vi "AppendEventInfoH5.vi"(6 "evt_num":i32, 8 "error in (no error)":errorcluster, 9 "evt_time":dbl, 10 "TDC Data":u32[](array[numeric]), 11 "dset in":T2 format="%.0x") -> (0 "error out":errorcluster)   [LabVIEW 2014]
uses:
  <vilib>/addons/h5labview2/base/hid_t.ctl
  <vilib>/addons/h5labview2/base/lib_path.vi
  <vilib>/addons/h5labview2/base/H5Equery.vi
  <vilib>/addons/h5labview2/dataset/H5Dwrite.llb/H5Dwrite.xnode
  <vilib>/addons/h5labview2/dataset/H5D.lvlib
  <vilib>/addons/h5labview2/space/H5S.lvlib
panel:
  in  "Cluster":T1
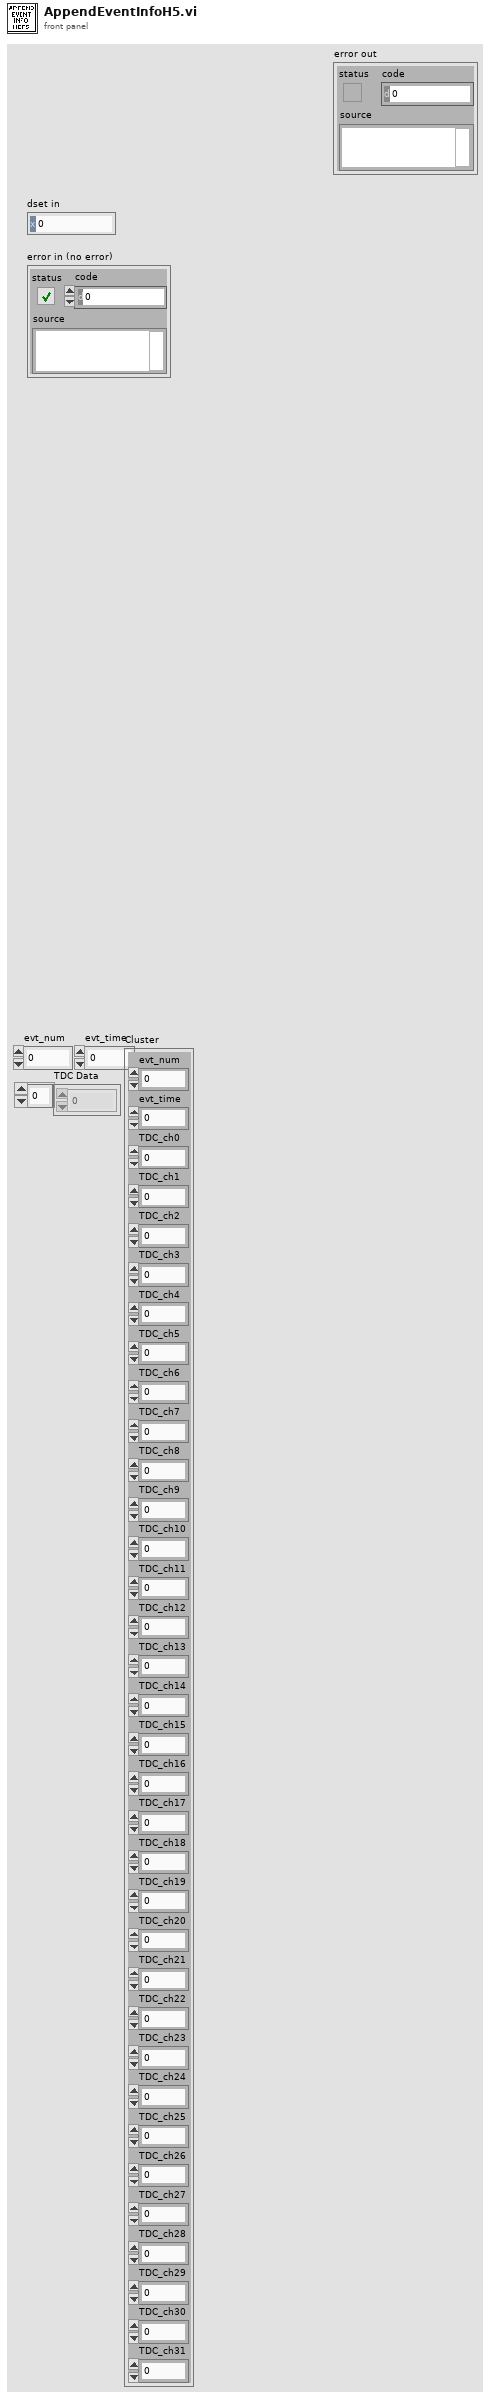
[diagram p1: front panel]
types:
  T1 = cluster{"evt_num":i32, "evt_time":dbl, "TDC_ch0":u32, "TDC_ch1":u32, "TDC_ch2":u32, "TDC_ch3":u32, "TDC_ch4":u32, "TDC_ch5":u32, "TDC_ch6":u32, "TDC_ch7":u32, "TDC_ch8":u32, "TDC_ch9":u32, "TDC_ch10":u32, "TDC_ch11":u32, "TDC_ch12":u32, "TDC_ch13":u32, "TDC_ch14":u32, "TDC_ch15":u32, "TDC_ch16":u32, "TDC_ch17":u32, "TDC_ch18":u32, "TDC_ch19":u32, "TDC_ch20":u32, "TDC_ch21":u32, "TDC_ch22":u32, "TDC_ch23":u32, "TDC_ch24":u32, "TDC_ch25":u32, "TDC_ch26":u32, "TDC_ch27":u32, "TDC_ch28":u32, "TDC_ch29":u32, "TDC_ch30":u32, "TDC_ch31":u32}
  T2 = typedef "hid_t.ctl" = i32
  T3 = cluster{"evt_num":i32, "evt_time":dbl, "TDC_ch0":u32, "TDC_ch1":u32, "TDC_ch2":u32, "TDC_ch3":u32, "TDC_ch4":u32, "TDC_ch5":u32, "TDC_ch6":u32, "TDC_ch7":u32, "TDC_ch8":u32, "TDC_ch9":u32, "TDC_ch10":u32, "TDC_ch11":u32, "TDC_ch12":u32, "TDC_ch13":u32, "TDC_ch14":u32, "TDC_ch15":u32, "TDC_ch16":u32, "TDC_ch17":u32, "TDC_ch18":u32, "TDC_ch19":u32, "TDC_ch20":u32, "TDC_ch21":u32, "TDC_ch22":u32, "TDC_ch23":u32, "TDC_ch24":u32, "TDC_ch25":u32, "TDC_ch26":u32, "TDC_ch27":u32, "TDC_ch28":u32, "TDC_ch29":u32, "TDC_ch30":u32, "TDC_ch31":u32}[]
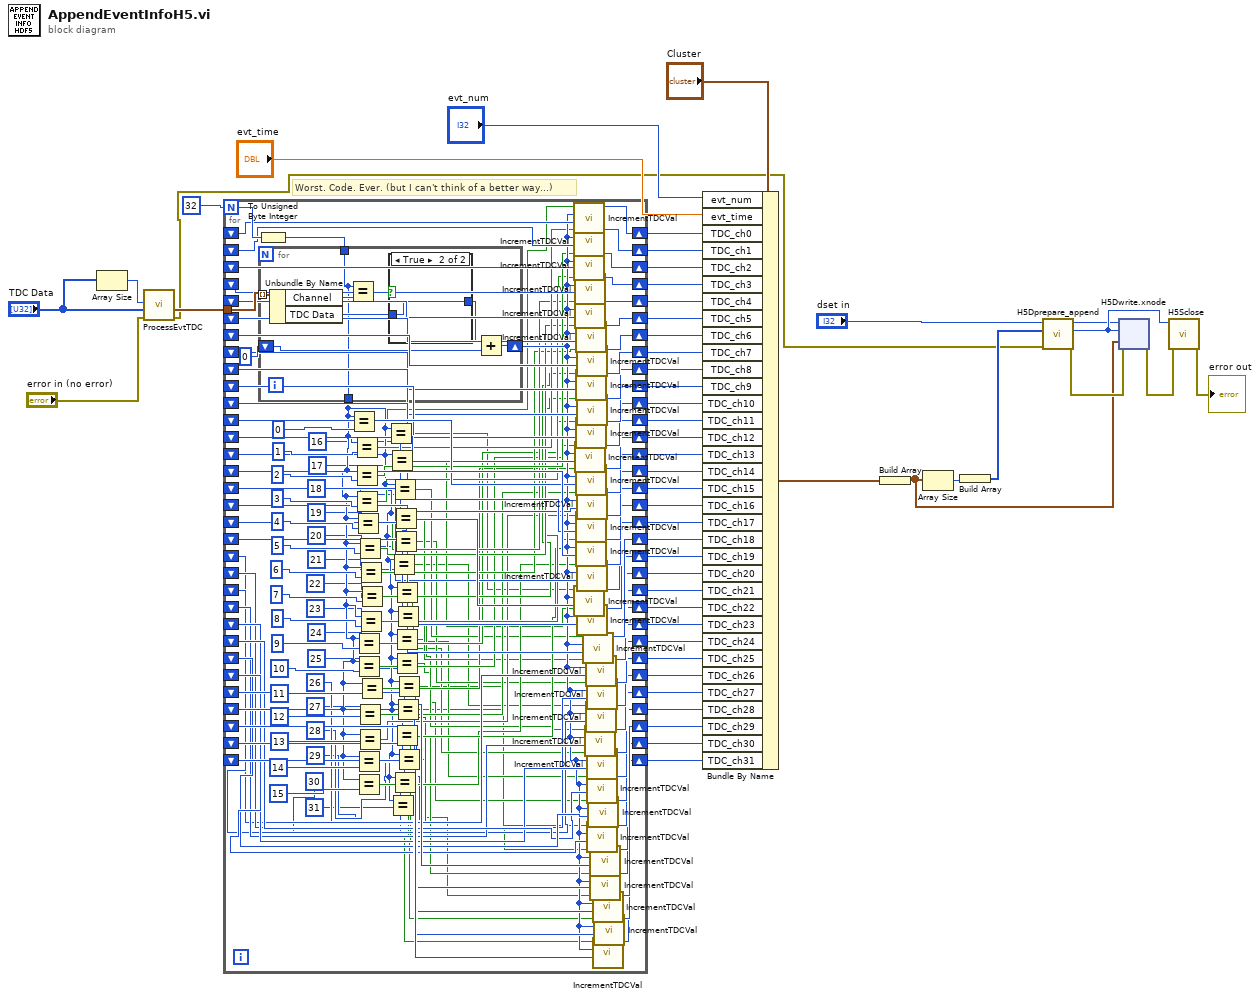
[diagram p0: block diagram]
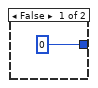
[diagram p2: hidden frame]
diagram:
  # "Worst. Code. Ever. (but I can't think of a better way...)"
  n1 = Array Size(array="TDC Data") -> (size(s)=w37:i32)
  n2 = call "ProcessEvtTDC.vi"("error in"="error in (no error)", "Encoded Data"="TDC Data", "# data points in evt"=w37) -> ("error out"=w1:errorcluster, "Decoded Data"=w34:cluster{"Channel":u8, "TDC Data":u16}[])  [unwired: 6 in, 1 out]
  n3 = for {
    N: u8 32 -> [w182]
    tunnel: w34 -> [w185]
    shift-right: [w180] -> w33
    shift-left: _ -> [w133]
    shift-right: [w179] -> w32
    shift-left: _ -> [w132]
    shift-right: [w177] -> w31
    shift-left: _ -> [w130]
    shift-right: [w176] -> w30
    shift-left: _ -> [w101]
    shift-right: [w175] -> w29
    shift-left: _ -> [w103]
    shift-right: [w174] -> w28
    shift-left: _ -> [w104]
    shift-right: [w173] -> w27
    shift-left: _ -> [w105]
    shift-right: [w172] -> w26
    shift-left: _ -> [w106]
    shift-right: [w171] -> w25
    shift-left: _ -> [w107]
    shift-right: [w170] -> w24
    shift-left: _ -> [w108]
    shift-right: [w169] -> w23
    shift-left: _ -> [w109]
    shift-right: [w178] -> w2
    shift-left: _ -> [w131]
    shift-right: [w168] -> w22
    shift-left: _ -> [w110]
    shift-right: [w167] -> w21
    shift-left: _ -> [w111]
    shift-right: [w166] -> w20
    shift-left: _ -> [w112]
    shift-right: [w165] -> w19
    shift-left: _ -> [w113]
    shift-right: [w164] -> w18
    shift-left: _ -> [w114]
    shift-right: [w163] -> w17
    shift-left: _ -> [w115]
    shift-right: [w162] -> w16
    shift-left: _ -> [w116]
    shift-right: [w161] -> w15
    shift-left: _ -> [w117]
    shift-right: [w160] -> w14
    shift-left: _ -> [w118]
    shift-right: [w159] -> w13
    shift-left: _ -> [w119]
    shift-right: [w158] -> w12
    shift-left: _ -> [w120]
    shift-right: [w157] -> w11
    shift-left: _ -> [w121]
    shift-right: [w156] -> w10
    shift-left: _ -> [w122]
    shift-right: [w155] -> w9
    shift-left: _ -> [w123]
    shift-right: [w154] -> w8
    shift-left: _ -> [w124]
    shift-right: [w153] -> w7
    shift-left: _ -> [w125]
    shift-right: [w152] -> w6
    shift-left: _ -> [w126]
    shift-right: [w151] -> w5
    shift-left: _ -> [w127]
    shift-right: [w150] -> w4
    shift-left: _ -> [w128]
    shift-right: [w149] -> w3
    shift-left: _ -> [w129]
    n4 = To Unsigned Byte Integer(number=w182) -> (unsigned 8bit integer=w184:u8)
    n5 = for {
      tunnel: w185 -> [w193] mode=indexing
      tunnel: w184 -> [w186]
      shift-right: [w189] -> w102
      shift-left: u16 0 ("TDC Data") -> [w188]
      tunnel: [w186] -> w84
      n6 = Unbundle By Name(w193) -> ("Channel"=w192:u8, "TDC Data"=w190:u16)
      n7 = Equal?(x=w186, y=w192) -> (x = y?=w191:bool)
      n8 = case shown="True" w191 {
        tunnel: w190 -> [_ w195]
        tunnel: [0 w195] -> w187
        frame False {
        }
        frame True {
        }
      }
      n9 = Add(x=w187, y=w188) -> (x+y=w189:i32)
    }
    n10 = Equal?(x=w84, y=0) -> (x = y?=w85:bool)
    n11 = Equal?(x=w84, y=1) -> (x = y?=w100:bool)
    n12 = Equal?(x=w84, y=2) -> (x = y?=w99:bool)
    n13 = Equal?(x=w84, y=3) -> (x = y?=w98:bool)
    n14 = Equal?(x=w84, y=4) -> (x = y?=w97:bool)
    n15 = Equal?(x=w84, y=9) -> (x = y?=w92:bool)
    n16 = Equal?(x=w84, y=10) -> (x = y?=w91:bool)
    n17 = Equal?(x=w84, y=14) -> (x = y?=w87:bool)
    n18 = Equal?(x=w84, y=15) -> (x = y?=w86:bool)
    n19 = Equal?(x=w84, y=5) -> (x = y?=w96:bool)
    n20 = Equal?(x=w84, y=12) -> (x = y?=w89:bool)
    n21 = Equal?(x=w84, y=13) -> (x = y?=w88:bool)
    n22 = Equal?(x=w84, y=6) -> (x = y?=w95:bool)
    n23 = Equal?(x=w84, y=8) -> (x = y?=w93:bool)
    n24 = Equal?(x=w84, y=7) -> (x = y?=w94:bool)
    n25 = Equal?(x=w84, y=11) -> (x = y?=w90:bool)
    n26 = Equal?(x=w84, y=16) -> (x = y?=w67:bool)
    n27 = Equal?(x=w84, y=17) -> (x = y?=w66:bool)
    n28 = Equal?(x=w84, y=31) -> (x = y?=w52:bool)
    n29 = Equal?(x=w84, y=21) -> (x = y?=w62:bool)
    n30 = Equal?(x=w84, y=18) -> (x = y?=w65:bool)
    n31 = Equal?(x=w84, y=30) -> (x = y?=w53:bool)
    n32 = Equal?(x=w84, y=19) -> (x = y?=w64:bool)
    n33 = Equal?(x=w84, y=20) -> (x = y?=w63:bool)
    n34 = Equal?(x=w84, y=22) -> (x = y?=w61:bool)
    n35 = Equal?(x=w84, y=24) -> (x = y?=w59:bool)
    n36 = Equal?(x=w84, y=25) -> (x = y?=w58:bool)
    n37 = Equal?(x=w84, y=28) -> (x = y?=w55:bool)
    n38 = Equal?(x=w84, y=23) -> (x = y?=w60:bool)
    n39 = Equal?(x=w84, y=27) -> (x = y?=w56:bool)
    n40 = Equal?(x=w84, y=26) -> (x = y?=w57:bool)
    n41 = Equal?(x=w84, y=29) -> (x = y?=w54:bool)
    n42 = call "IncrementTDCVal.vi"("val"=w133, "TDC Data"=w102, "Boolean"=w85) -> ("Numeric"=w180:i32)  [unwired: 8 in]
    n43 = call "IncrementTDCVal.vi"("val"=w132, "TDC Data"=w102, "Boolean"=w100) -> ("Numeric"=w179:i32)  [unwired: 8 in]
    n44 = call "IncrementTDCVal.vi"("val"=w131, "TDC Data"=w102, "Boolean"=w99) -> ("Numeric"=w178:i32)  [unwired: 8 in]
    n45 = call "IncrementTDCVal.vi"("val"=w114, "TDC Data"=w102, "Boolean"=w67) -> ("Numeric"=w164:i32)  [unwired: 8 in]
    n46 = call "IncrementTDCVal.vi"("val"=w130, "TDC Data"=w102, "Boolean"=w98) -> ("Numeric"=w177:i32)  [unwired: 8 in]
    n47 = call "IncrementTDCVal.vi"("val"=w101, "TDC Data"=w102, "Boolean"=w97) -> ("Numeric"=w176:i32)  [unwired: 8 in]
    n48 = call "IncrementTDCVal.vi"("val"=w108, "TDC Data"=w102, "Boolean"=w91) -> ("Numeric"=w170:i32)  [unwired: 8 in]
    n49 = call "IncrementTDCVal.vi"("val"=w103, "TDC Data"=w102, "Boolean"=w96) -> ("Numeric"=w175:i32)  [unwired: 8 in]
    n50 = call "IncrementTDCVal.vi"("val"=w105, "TDC Data"=w102, "Boolean"=w94) -> ("Numeric"=w173:i32)  [unwired: 8 in]
    n51 = call "IncrementTDCVal.vi"("val"=w107, "TDC Data"=w102, "Boolean"=w92) -> ("Numeric"=w171:i32)  [unwired: 8 in]
    n52 = call "IncrementTDCVal.vi"("val"=w109, "TDC Data"=w102, "Boolean"=w90) -> ("Numeric"=w169:i32)  [unwired: 8 in]
    n53 = call "IncrementTDCVal.vi"("val"=w111, "TDC Data"=w102, "Boolean"=w88) -> ("Numeric"=w167:i32)  [unwired: 8 in]
    n54 = call "IncrementTDCVal.vi"("val"=w112, "TDC Data"=w102, "Boolean"=w87) -> ("Numeric"=w166:i32)  [unwired: 8 in]
    n55 = call "IncrementTDCVal.vi"("val"=w104, "TDC Data"=w102, "Boolean"=w95) -> ("Numeric"=w174:i32)  [unwired: 8 in]
    n56 = call "IncrementTDCVal.vi"("val"=w106, "TDC Data"=w102, "Boolean"=w93) -> ("Numeric"=w172:i32)  [unwired: 8 in]
    n57 = call "IncrementTDCVal.vi"("val"=w110, "TDC Data"=w102, "Boolean"=w89) -> ("Numeric"=w168:i32)  [unwired: 8 in]
    n58 = call "IncrementTDCVal.vi"("val"=w113, "TDC Data"=w102, "Boolean"=w86) -> ("Numeric"=w165:i32)  [unwired: 8 in]
    n59 = call "IncrementTDCVal.vi"("val"=w115, "TDC Data"=w102, "Boolean"=w66) -> ("Numeric"=w163:i32)  [unwired: 8 in]
    n60 = call "IncrementTDCVal.vi"("val"=w116, "TDC Data"=w102, "Boolean"=w65) -> ("Numeric"=w162:i32)  [unwired: 8 in]
    n61 = call "IncrementTDCVal.vi"("val"=w120, "TDC Data"=w102, "Boolean"=w61) -> ("Numeric"=w158:i32)  [unwired: 8 in]
    n62 = call "IncrementTDCVal.vi"("val"=w117, "TDC Data"=w102, "Boolean"=w64) -> ("Numeric"=w161:i32)  [unwired: 8 in]
    n63 = call "IncrementTDCVal.vi"("val"=w119, "TDC Data"=w102, "Boolean"=w62) -> ("Numeric"=w159:i32)  [unwired: 8 in]
    n64 = call "IncrementTDCVal.vi"("val"=w118, "TDC Data"=w102, "Boolean"=w63) -> ("Numeric"=w160:i32)  [unwired: 8 in]
    n65 = call "IncrementTDCVal.vi"("val"=w121, "TDC Data"=w102, "Boolean"=w60) -> ("Numeric"=w157:i32)  [unwired: 8 in]
    n66 = call "IncrementTDCVal.vi"("val"=w122, "TDC Data"=w102, "Boolean"=w59) -> ("Numeric"=w156:i32)  [unwired: 8 in]
    n67 = call "IncrementTDCVal.vi"("val"=w124, "TDC Data"=w102, "Boolean"=w57) -> ("Numeric"=w154:i32)  [unwired: 8 in]
    n68 = call "IncrementTDCVal.vi"("val"=w123, "TDC Data"=w102, "Boolean"=w58) -> ("Numeric"=w155:i32)  [unwired: 8 in]
    n69 = call "IncrementTDCVal.vi"("val"=w125, "TDC Data"=w102, "Boolean"=w56) -> ("Numeric"=w153:i32)  [unwired: 8 in]
    n70 = call "IncrementTDCVal.vi"("val"=w126, "TDC Data"=w102, "Boolean"=w55) -> ("Numeric"=w152:i32)  [unwired: 8 in]
    n71 = call "IncrementTDCVal.vi"("val"=w127, "TDC Data"=w102, "Boolean"=w54) -> ("Numeric"=w151:i32)  [unwired: 8 in]
    n72 = call "IncrementTDCVal.vi"("val"=w129, "TDC Data"=w102, "Boolean"=w52) -> ("Numeric"=w149:i32)  [unwired: 8 in]
    n73 = call "IncrementTDCVal.vi"("val"=w128, "TDC Data"=w102, "Boolean"=w53) -> ("Numeric"=w150:i32)  [unwired: 8 in]
  }
  n74 = Bundle By Name(cluster="Cluster", "evt_num"="evt_num", "evt_time"="evt_time", "TDC_ch0"=w33, "TDC_ch1"=w32, "TDC_ch2"=w2, "TDC_ch3"=w31, "TDC_ch4"=w30, "TDC_ch5"=w29, "TDC_ch6"=w28, "TDC_ch7"=w27, "TDC_ch8"=w26, "TDC_ch9"=w25, "TDC_ch10"=w24, "TDC_ch11"=w23, "TDC_ch12"=w22, "TDC_ch13"=w21, "TDC_ch14"=w20, "TDC_ch15"=w19, "TDC_ch16"=w18, "TDC_ch17"=w17, "TDC_ch18"=w16, "TDC_ch19"=w15, "TDC_ch20"=w14, "TDC_ch21"=w13, "TDC_ch22"=w12, "TDC_ch23"=w11, "TDC_ch24"=w10, "TDC_ch25"=w9, "TDC_ch26"=w8, "TDC_ch27"=w7, "TDC_ch28"=w6, "TDC_ch29"=w5, "TDC_ch30"=w4, "TDC_ch31"=w3) -> (w41:T1)
  n75 = Build Array(w41) -> (w43:T3)
  n76 = Array Size(array=w43) -> (size(s)=w45:i32)
  n77 = Build Array(w45) -> (w44:i32[])
  n78 = call <vilib>:"H5Dprepare_append.vi"("error in (no error)"=w1, "append dims"=w44, "dset in"="dset in") -> ("error out"=w48:errorcluster, "space out"=w50:T2, "dset out"=w49:T2)  [unwired: 6 in]
  n79 = xnode "H5Dwrite.xnode"("error in (no error)"=w48, "data"=w43, "file space"=w50, "ref in"=w49) -> ("error out"=w51:errorcluster)  [unwired: 3 in, 2 out]
  n80 = call <vilib>:"H5Sclose.vi"("error in (no error)"=w51, "space in"=w50) -> ("error out"=→"error out":errorcluster)  [unwired: 9 in]
